vi "Get DIO Port A, B, C direction.vi"(8 "error in (no error)":errorcluster, 11 "VISA resource name":refnum<visa-resource-name>) -> (0 "error out":errorcluster, 2 "Port A, B direction":T1, 3 "VISA resource name out":refnum<visa-resource-name>)   [LabVIEW 2014, in "Newport ESP301.lvlib"]
doc: "This command is used to get digital I/O (DIO) port A and B direction where bit-0\ncorresponds to port A and B, bit-1 to port B. If any bit is set to zero(0) then its\ncorresponding port will become an input only. If any bit is set to one(1) then its\ncorresponding port will becomes an output only.\nA DIO within a port configured as an input can only report its present HIGH or\nLOW logic level. Whereas a DIO bit within a port configured as an output can\nset(1) or clear(0) the corresponding DIO hardware to HIGH or LOW logic level.\nReading the status of a port configured as output returns its present output status.\nNOTE: All direction bits are automatically zeroed, or cleared, after a system\nreset. Therefore all DIO ports default to input by default.\nNOTE: Each DIO bit has a pulled-up resistor to +5V. Therefore, all bits will be\nat HIGH logic level if not connected to external circuit and configured as input."
uses:
  Newport ESP301.lvlib
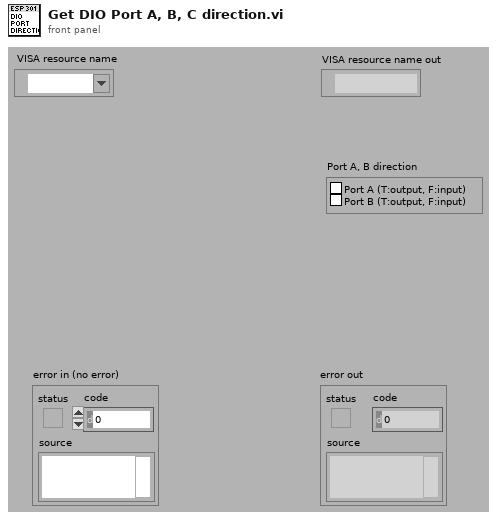
[diagram p1: front panel]
types:
  T1 = cluster{"Port A (T:output, F:input)":bool, "Port B (T:output, F:input)":bool}
  T2 = cluster{"Boolean array[0]":bool, "Boolean array[1]":bool}
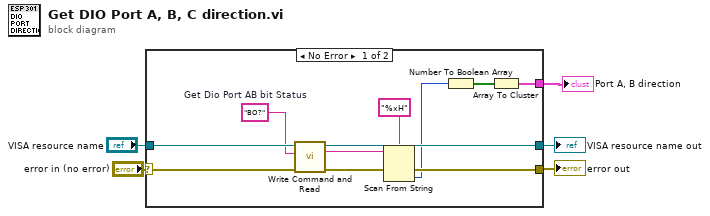
[diagram p0: block diagram]
diagram:
  n1 = case shown="No Error" "error in (no error)" {
    selector: "error in (no error)" -> [w14 w18]
    tunnel: [w10 w18] -> w3
    tunnel: "VISA resource name" -> [w16 w17]
    tunnel: [w15 w17] -> w2
    tunnel: [w7 _] -> w1
    frame No Error {
      w13 = "BO?"  # Get Dio Port AB bit Status
      n2 = call "Write Command and Read.vi"("error in (no error)"=w14, "Command"=w13, "VISA resource name"=w16) -> ("error out"=w11:errorcluster, "Returned string"=w9:string, "VISA resource name out"=w15:refnum<visa-resource-name>)  [unwired: 2 in, 2 out]
      n3 = Scan From String(format string="%xH" ("chaîne de format"), input string=w9, error in=w11) -> (error out=w10:errorcluster, output 1=w8:u32)  [unwired: 2 in, 2 out]
      n4 = Number To Boolean Array(number=w8) -> (Boolean array=w12:bool[])
      n5 = Array To Cluster(array=w12) -> (cluster=w7:T2)
    }
    frame Error {
    }
  }
  "error out" <- w3
  "VISA resource name out" <- w2
  "Port A, B direction" <- w1
